vi "Sync.Start.vi"(8 "error in":errorcluster, 11 "DAQmx in":refnum<class "DAQmx.lvclass">) -> (0 "error out":errorcluster, 3 "DAQmx out":refnum<class "DAQmx.lvclass">)   [LabVIEW 2019, in "DAQmx.lvclass"]
uses:
  DAQmx.lvclass
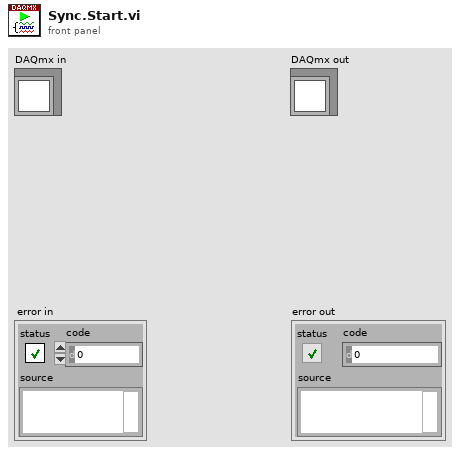
[diagram p1: front panel]
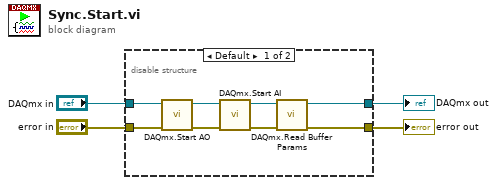
[diagram p0: block diagram]
diagram:
  n1 = disable-structure shown="Default" {
    disable-tunnel: "DAQmx in" -> [w10 w14]
    disable-tunnel: "error in" -> [w9 w13]
    disable-tunnel: [w6 w14] -> w3
    disable-tunnel: [w5 w13] -> w2
    frame condition #0 (active) {
      n2 = call "DAQmx.Start AO.vi"("error in (no error)"=w9, "DAQmx in"=w10) -> ("error out"=w12:errorcluster, "DAQmx out"=w11:refnum<class "DAQmx.lvclass">)  [unwired: 8 in]
      n3 = call "DAQmx.Start AI.vi"("error in (no error)"=w12, "DAQmx in"=w11) -> ("error out"=w8:errorcluster, "DAQmx out"=w7:refnum<class "DAQmx.lvclass">)  [unwired: 6 in]
      n4 = call "DAQmx.Read Buffer Params.vi"("error in (no error)"=w8, "DAQmx in"=w7) -> ("error out"=w5:errorcluster, "DAQmx out"=w6:refnum<class "DAQmx.lvclass">)  [unwired: 8 in]
    }
    frame condition #1 {
    }
  }
  "error out" <- w2
  "DAQmx out" <- w3
